vi "pallet DB.vi"(0 "pallet_num":i32, 1 "connection reference":T1, 2 "info array":dbl[][](array[numeric]), 4 "Table":string="disc10", 6 "set data":bool, 9 "error in":errorcluster) -> (23 "connection reference out":T1, 27 "error out":errorcluster)   [LabVIEW 2019]
uses:
  <vilib>/addons/database/Connection.llb/Conn ObjectReference.ctl
  <vilib>/addons/database/Auxilliary.llb/DB Tools Format Datetime String (Time Stamp).vi
  <vilib>/addons/database/NI_Database_API.lvlib
panel:
  in  "Numeric":i32
  # "Database table"
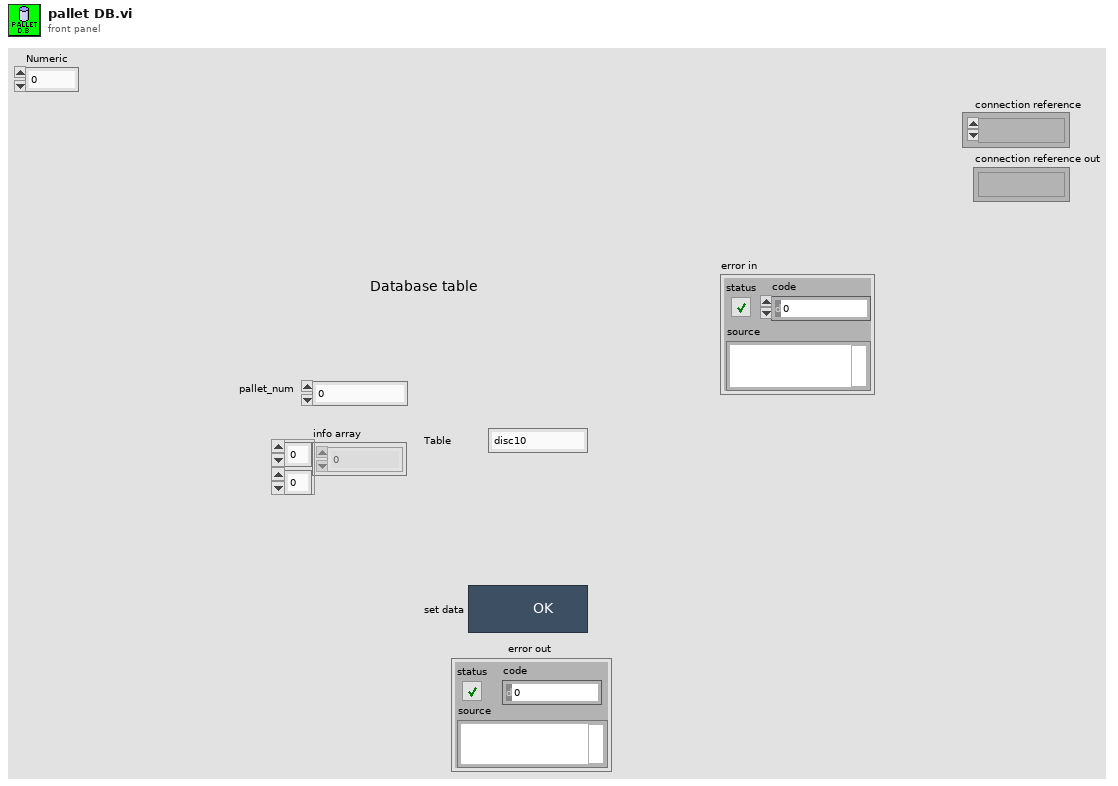
[diagram p1: front panel]
types:
  T1 = typedef "NI_Database_API.lvlib/Conn ObjectReference.ctl" = refnum<k1>
  T2 = cluster{string, "date/time string":string, string, string, string, string, string, string, string, string, string, string, string, string, string, "Numeric":i32}
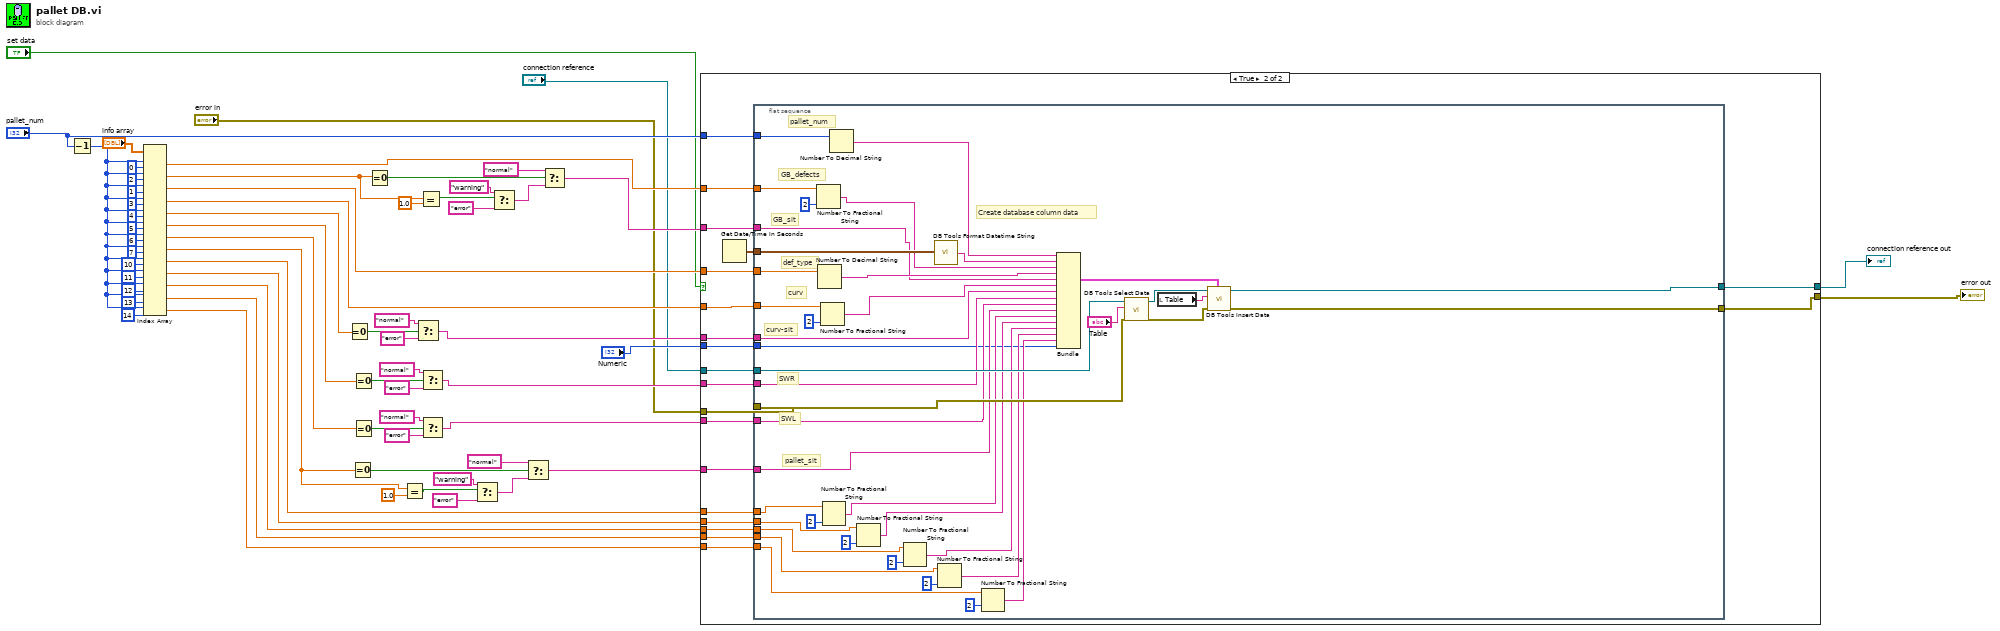
[diagram p0: block diagram]
diagram:
  n1 = Decrement(x="pallet_num") -> (x-1=w17:i32)
  n2 = Index Array(array="info array", index (row) #1=w17, index (col) #1=0 ("disabled index (col)"), index (row) #2=w17, index (col) #2=2 ("disabled index (col)"), index (row) #3=w17, index (col) #3=1 ("disabled index (col)"), index (row) #4=w17, index (col) #4=3 ("disabled index (col)"), index (row) #5=w17, index (col) #5=4 ("disabled index (col)"), index (row) #6=w17, index (col) #6=5 ("disabled index (col)"), index (row) #7=w17, index (col) #7=6 ("disabled index (col)"), index (row) #8=w17, index (col) #8=7 ("disabled index (col)"), index (row) #9=w17, index (col) #9=10 ("disabled index (col)"), index (row) #10=w17, index (col) #10=11 ("disabled index (col)"), index (row) #11=w17, index (col) #11=12 ("disabled index (col)"), index (row) #12=w17, index (col) #12=13 ("disabled index (col)"), index (row) #13=w17, index (col) #13=14 ("disabled index (col)")) -> (element #1=w54:dbl, element #2=w48:dbl, element #3=w53:dbl, element #4=w43:dbl, element #5=w42:dbl, element #6=w31:dbl, element #7=w30:dbl, element #8=w19:dbl, element #9=w11:dbl, element #10=w10:dbl, element #11=w9:dbl, element #12=w8:dbl, element #13=w7:dbl)
  n3 = Equal To 0?(x=w42) -> (x = 0?=w41:bool)
  n4 = Equal To 0?(x=w19) -> (x = 0?=w20:bool)
  n5 = Equal To 0?(x=w31) -> (x = 0?=w35:bool)
  n6 = Equal To 0?(x=w30) -> (x = 0?=w34:bool)
  n7 = Equal To 0?(x=w48) -> (x = 0?=w52:bool)
  n8 = Equal?(x=w19, y=1.0) -> (x = y?=w25:bool)
  n9 = Select(t="normal", s=w41, f="error") -> (s? t:f=w38:string)
  n10 = Equal?(x=w48, y=1.0) -> (x = y?=w46:bool)
  n11 = Select(t="normal", s=w35, f="error") -> (s? t:f=w29:string)
  n12 = Select(t="normal", s=w34, f="error") -> (s? t:f=w28:string)
  n13 = Select(t="warning", s=w25, f="error") -> (s? t:f=w26:string)
  n14 = Select(t="warning", s=w46, f="error") -> (s? t:f=w45:string)
  n15 = Select(t="normal", s=w20, f=w26) -> (s? t:f=w18:string)
  n16 = Select(t="normal", s=w52, f=w45) -> (s? t:f=w44:string)
  n17 = case shown="True" "set data" {
    tunnel: "error in" -> [w65 w85]
    tunnel: [w65 w83] -> w1
    tunnel: [w64 w82] -> w3
    tunnel: "connection reference" -> [w64 w81]
    tunnel: "pallet_num" -> [_ w80]
    tunnel: w54 -> [_ w79]
    tunnel: w53 -> [_ w78]
    tunnel: w44 -> [_ w77]
    tunnel: w43 -> [_ w76]
    tunnel: w38 -> [_ w75]
    tunnel: w29 -> [_ w74]
    tunnel: w28 -> [_ w73]
    tunnel: w18 -> [_ w72]
    tunnel: w11 -> [_ w71]
    tunnel: w10 -> [_ w70]
    tunnel: w9 -> [_ w69]
    tunnel: w8 -> [_ w68]
    tunnel: w7 -> [_ w67]
    tunnel: "Numeric" -> [_ w66]
    frame False {
    }
    frame True {
      n18 = Get Date/Time In Seconds() -> (seconds since 1Jan1904=w84:timestamp)
      n19 = flat-sequence {
        tunnel: [w86] -> w83
        tunnel: [w87] -> w82
        tunnel: w66 -> [w88]
        tunnel: w67 -> [w99]
        tunnel: w68 -> [w100]
        tunnel: w69 -> [w101]
        tunnel: w70 -> [w102]
        tunnel: w71 -> [w103]
        tunnel: w72 -> [w106]
        tunnel: w73 -> [w107]
        tunnel: w74 -> [w108]
        tunnel: w75 -> [w109]
        tunnel: w76 -> [w110]
        tunnel: w77 -> [w104]
        tunnel: w78 -> [w111]
        tunnel: w79 -> [w112]
        tunnel: w80 -> [w113]
        tunnel: w81 -> [w115]
        tunnel: w84 -> [w121]
        tunnel: w85 -> [w114]
        frame #0 {
          # "pallet_sit"
          # "SWL"
          # "SWR"
          # "curv-sit"
          # "curv"
          # "def_type"
          # "GB_sit"
          # "GB_defects"
          # "pallet_num"
          # "Create database column data"
          n20 = Number To Fractional String(number=w112, precision (6)=i16 2) -> (F-format string=w119:string)  [unwired: 2 in]
          n21 = Number To Decimal String(number=w111) -> (decimal integer string=w105:string)  [unwired: 1 in]
          n22 = Number To Fractional String(number=w110, precision (6)=i16 2) -> (F-format string=w116:string)  [unwired: 2 in]
          n23 = Number To Fractional String(number=w103, precision (6)=i16 2) -> (F-format string=w93:string)  [unwired: 2 in]
          n24 = Number To Decimal String(number=w113) -> (decimal integer string=w120:string)  [unwired: 1 in]
          n25 = Number To Fractional String(number=w102, precision (6)=i16 2) -> (F-format string=w92:string)  [unwired: 2 in]
          n26 = Number To Fractional String(number=w101, precision (6)=i16 2) -> (F-format string=w91:string)  [unwired: 2 in]
          n27 = call-poly <vilib>:"DB Tools Format Datetime String.vi"("time stamp"=w121) -> ("date/time string"=w123:string)
          n28 = Number To Fractional String(number=w100, precision (6)=i16 2) -> (F-format string=w90:string)  [unwired: 2 in]
          n29 = Number To Fractional String(number=w99, precision (6)=i16 2) -> (F-format string=w89:string)  [unwired: 2 in]
          n30 = Bundle(w120, "date/time string"=w123, w119, w105, w104, w116, w109, w108, w107, w106, w93, w92, w91, w90, w89, "Numeric"=w88) -> (w122:T2)  [unwired: 1 in]
          n31 = call <vilib>:"DB Tools Select Data.vi"("error in (no error)"=w114, "table"="Table", "connection reference"=w115) -> ("error out"=w125:errorcluster, "connection reference out"=w126:T1)  [unwired: 3 in, 1 out]
          n32 = local read "Table"() -> (w127:string)
          n33 = call <vilib>:"DB Tools Insert Data.vi"("data"=w122, "error in (no error)"=w125, "table"=w127, "connection reference"=w126) -> ("error out"=w86:errorcluster, "connection reference out"=w87:T1)  [unwired: 6 in]
        }
      }
    }
  }
  "error out" <- w1
  "connection reference out" <- w3
